vi "lab5.vi"() -> ()   [LabVIEW 2018]
panel:
  in  "type":enum16{"Simulation module", "Euler (recursive)"}(ring)
  in  "конец по времени":dbl=30.0
  in  "шаг по времени":dbl=0.01
  out "result":cluster{dbl[], dbl[]}(graph)
  in  "a":dbl=0.00517028
  in  "step":dbl=0.01
  in  "start":dbl=0.1
  in  "Array":dbl[][](array[numeric])=[[-9.69284, -65.7276, -204.821], [1.0, 0.0, 0.0], [0.0, 1.0, 0.0]]
  in  "end":dbl=10.0
  # "начальная частота"
  # "x'=-cx-dy-bz+1\ny'=x\nz'=y\nout = ax+bz"
  # "шаг по частоте"
  # "конечная частота"
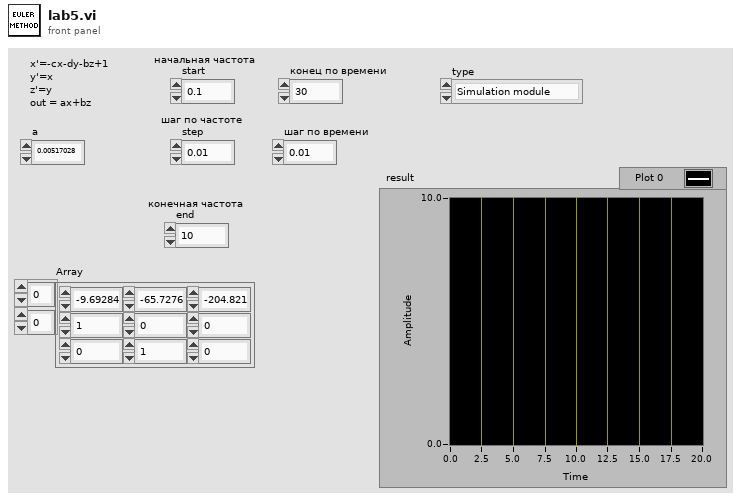
[diagram p1: front panel]
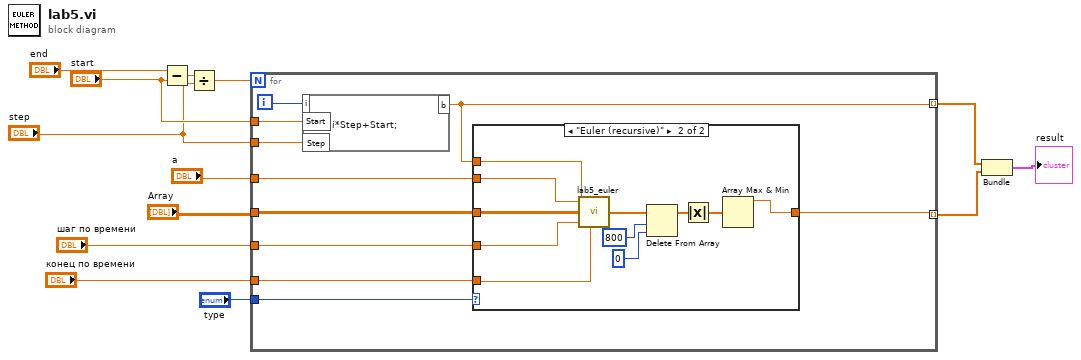
[diagram p0: block diagram]
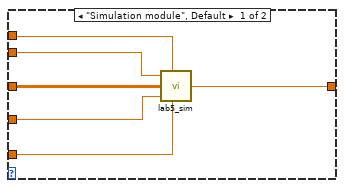
[diagram p2: hidden frame]
diagram:
  n1 = Subtract(x="end", y="start") -> (x-y=w10:dbl)
  n2 = Divide(x=w10, y="step") -> (x/y=w1:dbl)
  n3 = for {
    N: w1 -> [_]
    tunnel: [w14] -> w13 mode=indexing
    tunnel: [w15] -> w12 mode=indexing
    tunnel: "start" -> [w22]
    tunnel: "step" -> [w16]
    tunnel: "шаг по времени" -> [w19]
    tunnel: "конец по времени" -> [w17]
    tunnel: "a" -> [w18]
    tunnel: "Array" -> [w20]
    tunnel: "type" -> [w21]
    i -> [w23]
    n4 = formula code="b = i*Step+Start;"("i"=w23, "Start"=w22, "Step"=w16) -> ("b"=w15:dbl)
    n5 = case shown="\"Euler (recursive)\"" w21 {
      tunnel: w20 -> [w27 w38]
      tunnel: w19 -> [w26 w37]
      tunnel: w18 -> [w28 w39]
      tunnel: w17 -> [w25 w36]
      tunnel: w15 -> [w29 w40]
      tunnel: [w24 w30] -> w14
      frame "Simulation module", Default {
        n6 = call "lab5_sim.vi"("какая-то константа для ответа"=w28, "считаем в цикле"=w29, "Array"=w27, "шаг по времени"=w26, "конец по времени"=w25) -> ("res"=w24:dbl)
      }
      frame "Euler (recursive)" {
        n7 = call "lab5_euler.vi"("a"=w39, "b"=w40, "Array"=w38, "шаг по времени"=w37, "конец по времени"=w36) -> ("Array out"=w31:dbl[])
        n8 = Delete From Array(array=w31, length=800, index=0) -> (array with subset deleted=w33:dbl[])  [unwired: 1 out]
        n9 = Absolute Value(x=w33) -> (abs(x)=w32:dbl[])
        n10 = Array Max & Min(array=w32) -> (max value=w30:dbl)  [unwired: 3 out]
      }
    }
  }
  n11 = Bundle "Bundle"(w12, w13) -> (→"result":cluster{dbl[], dbl[]})  [unwired: 1 in]
